vi "Canceled.vi"(8 "error in (no error)":errorcluster, 9 "Timeout (0)":i32, 11 "Bar in":refnum<class "Bar.lvclass">) -> (0 "error out":errorcluster, 2 "Canceled by user?":bool, 3 "Bar out":refnum<class "Bar.lvclass">)   [LabVIEW 2015, in "Simple Progress Bar.lvlib" / "Bar.lvclass"]
uses:
  Bar.lvclass
  Bar.lvclass/Bar.ctl
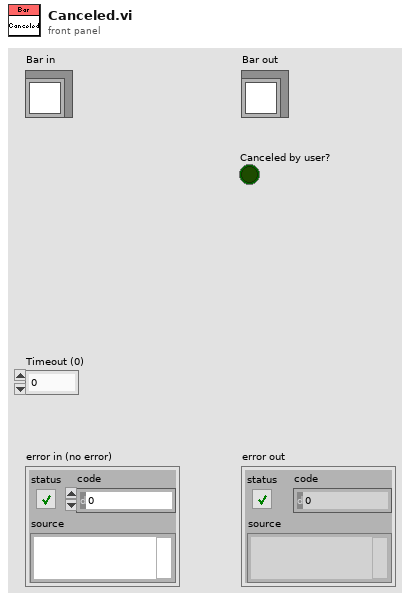
[diagram p1: front panel]
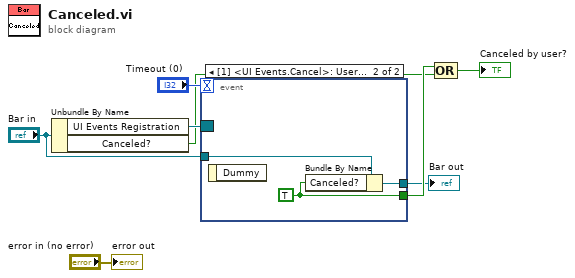
[diagram p0: block diagram]
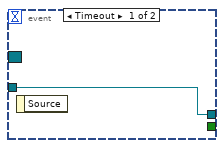
[diagram p2: hidden frame]
diagram:
  n1 = Unbundle By Name("Bar in") -> ("UI Events Registration"=w5:refnum<event-registration>, "Canceled?"=w1:bool)
  n2 = event shown="[1] <UI Events.Cancel>: User Event" {
    selector: w5 -> [_ _]
    dyn-events: _ -> [_ _]
    timeout: "Timeout (0)" -> [_ _]
    tunnel: [_ w10] -> w8
    tunnel: "Bar in" -> [w9 w12]
    tunnel: [w9 w11] -> w3
    event Timeout {
      n3 = event-data() -> ()  [unwired: 1 in, 1 out]
    }
    event User Event {
      w10 = TRUE
      n4 = event-data() -> ()  [unwired: 1 in, 1 out]
      n5 = Bundle By Name(cluster=w12, "Canceled?"=w10) -> (w11:refnum<class "Bar.lvclass">)
    }
  }
  "Bar out" <- w3
  n6 = Compound Arithmetic op=OR(w8, w1) -> (→"Canceled by user?":bool)
  "error out" <- "error in (no error)"
